vi "createEvents.vi"(8 "error in (no error)":errorcluster, 11 "CameraEventsManger in":refnum<class "CameraEventsManger.lvclass">) -> (0 "error out":errorcluster, 3 "CameraEventsManger out":refnum<class "CameraEventsManger.lvclass">)   [LabVIEW 2009, in "Tools.lvlib" / "Settings.lvlib" / "CameraEventsManger.lvclass"]
uses:
  CameraEventsManger.lvclass
  Viewers/Snapper/SnapperEvents.lvclass
  Tools/SettingsEventManager/SettingsEventsManager.lvclass
  CameraEventsManger.lvclass/CameraEventsManger.ctl
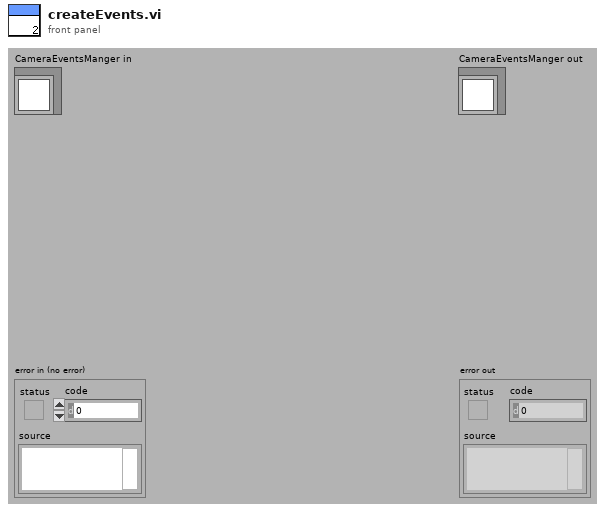
[diagram p1: front panel]
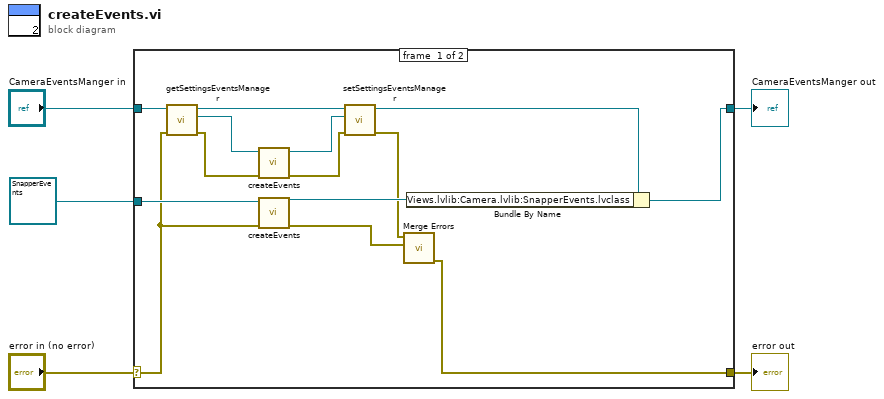
[diagram p0: block diagram]
diagram:
  n1 = case shown="No Error" "error in (no error)" {
    selector: "error in (no error)" -> [w12 w21]
    tunnel: [w6 w21] -> w4
    tunnel: [w10 w20] -> w2
    tunnel: "CameraEventsManger in" -> [w19 w20]
    tunnel: refnum<class "SnapperEvents.lvclass"> refnum ("Views.lvlib:Camera.lvlib:SnapperEvents.lvclass") -> [w13 _]
    frame #0 {
      n2 = call-dynamic "getSettingsEventsManager.vi"("error in (no error)"=w12, "CameraEventsManger.lvclass in"=w19) -> ("error out"=w17:errorcluster, "SettingsEventsManager"=w18:refnum<class "SettingsEventsManager.lvclass">, "CameraEventsManger.lvclass out"=w16:refnum<class "CameraEventsManger.lvclass">)  [unwired: 7 in]
      n3 = call-dynamic "createEvents.vi"("error in (no error)"=w17, "SettingsEventsManager in"=w18) -> ("error out"=w14:errorcluster, "SettingsEventsManager out"=w15:refnum<class "SettingsEventsManager.lvclass">)  [unwired: 8 in]
      n4 = call-dynamic "createEvents.vi"("error in (no error)"=w12, "SnapperEvents in"=w13) -> ("error out"=w8:errorcluster, "SnapperEvents out"=w9:refnum<class "SnapperEvents.lvclass">)  [unwired: 8 in]
      n5 = call-dynamic "setSettingsEventsManager.vi"("error in (no error)"=w14, "Tools.lvlib:Settings.lvlib:SettingsEventsManager.lvclass"=w15, "CameraEventsManger.lvclass in"=w16) -> ("error out"=w7:errorcluster, "CameraEventsManger.lvclass out"=w11:refnum<class "CameraEventsManger.lvclass">)  [unwired: 7 in]
      n6 = call <vilib>:"Merge Errors.vi"("error in 2 (no error)"=w8, "error in 1 (no error)"=w7) -> ("error out"=w6:errorcluster)  [unwired: 5 in]
      n7 = Bundle By Name(cluster=w11, "Views.lvlib:Camera.lvlib:SnapperEvents.lvclass"=w9) -> (w10:refnum<class "CameraEventsManger.lvclass">)
    }
    frame #1 {
    }
  }
  "error out" <- w4
  "CameraEventsManger out" <- w2
